vi "increment Modbus address.vi"(0 "available addresses":T1(array[cluster]), 1 "string length":i32, 5 "modbus type":T2, 7 "data type":T3) -> (4 "available addresses out":T1(array[cluster]), 6 "starting address":u16, 8 "subindex (bool)":i32)   [LabVIEW 2013, in "Modbus Module configuration.lvclass"]
uses:
  Modbus Module configuration.lvclass
  <vilib>/NI/Tag Bus/tag/Data Type.ctl
  module channel/data bank type.ctl
  <vilib>/NI/Tag Bus/tag/tag descriptor.lvclass
  module channel/Modbus Module Channel.lvclass
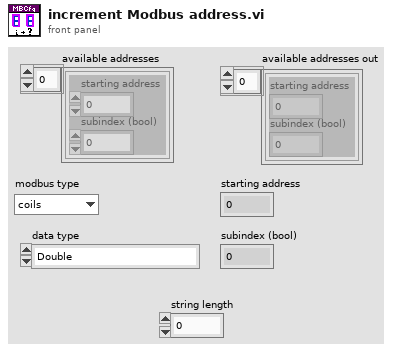
[diagram p1: front panel]
types:
  T1 = cluster{"starting address":u16, "subindex (bool)":i32}[]
  T2 = typedef "Modbus Module Channel.lvclass/data bank type.ctl" = enum16{"coils", "discrete inputs", "input registers", "holding registers"}
  T3 = typedef "tag bus.lvlib/tag descriptor.lvclass/Data Type.ctl" = enum16{"Double", "Single", "I64", "I32", "I16", "I8", "U64", "U32", "U16", "U8", "Boolean", "String", "Array of Double", "Array of Single", "Array of I64", "Array of I32", "Array of I16", "Array of I8", "Array of U64", "Array of U32", "Array of U16", "Array of U8", "Array of Boolean", "Array of String"}
  T4 = cluster{"starting address":u16, "subindex (bool)":i32}
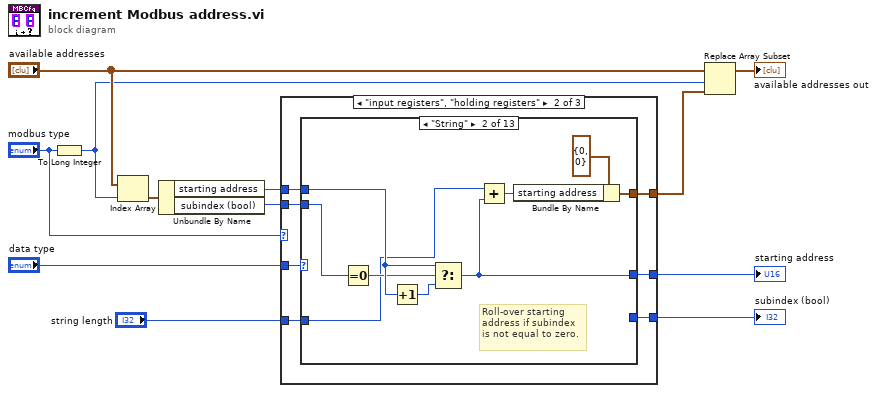
[diagram p0: block diagram]
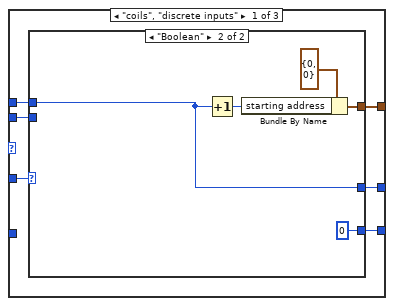
[diagram p2: hidden frame]
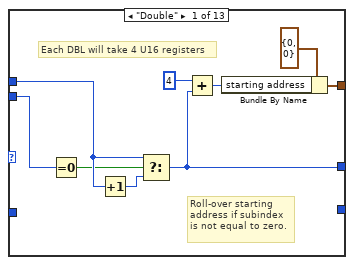
[diagram p4: hidden frame]
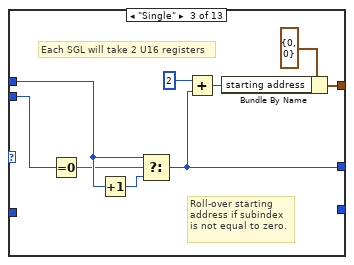
[diagram p5: hidden frame]
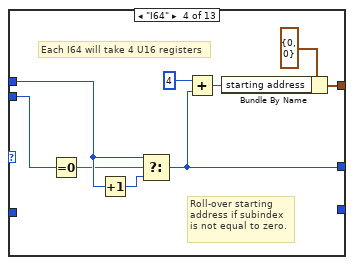
[diagram p6: hidden frame]
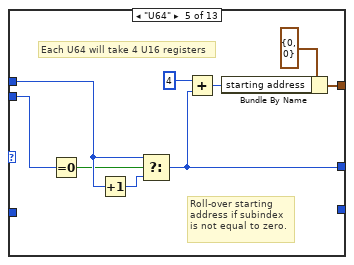
[diagram p7: hidden frame]
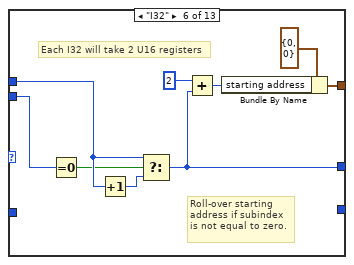
[diagram p8: hidden frame]
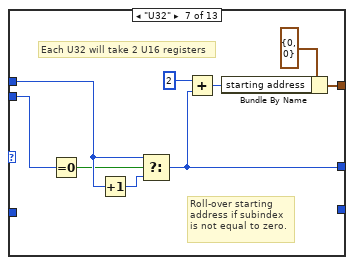
[diagram p9: hidden frame]
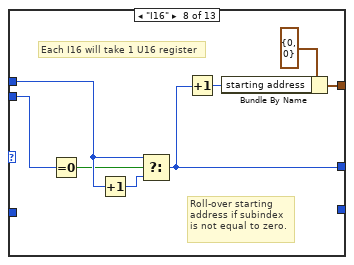
[diagram p10: hidden frame]
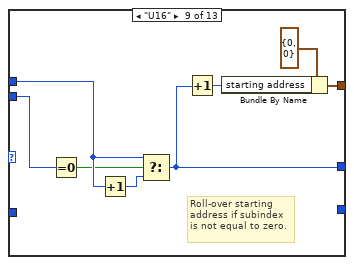
[diagram p11: hidden frame]
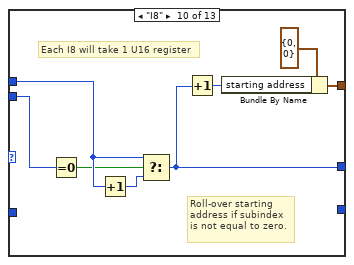
[diagram p12: hidden frame]
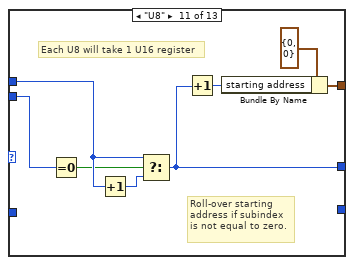
[diagram p13: hidden frame]
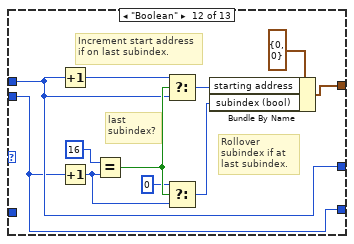
[diagram p14: hidden frame]
diagram:
  n1 = To Long Integer(number="modbus type") -> (32bit integer=w9:i32)
  n2 = Index Array(array="available addresses", index=w9) -> (element=w11:T4)
  n3 = Unbundle By Name(w11) -> ("starting address"=w5:u16, "subindex (bool)"=w8:i32)
  n4 = case shown="\"input registers\", \"holding registers\"" "modbus type" {
    tunnel: "data type" -> [w18 w30 _]
    tunnel: w8 -> [w17 w29 _]
    tunnel: [w16 w28 _] -> w6
    tunnel: w5 -> [w15 w27 _]
    tunnel: [w14 w26 _] -> w4
    tunnel: [w13 w25 _] -> w3
    tunnel: "string length" -> [_ w24 _]
    frame "coils", "discrete inputs" {
      n5 = case shown="\"Boolean\"" w18 {
        tunnel: w17 -> [_ _]
        tunnel: w15 -> [_ w19]
        tunnel: [_ w22] -> w16
        tunnel: [_ w19] -> w14
        tunnel: [_ 0 ("subindex (bool)")] -> w13
        frame Default {
        }
        frame "Boolean" {
          n6 = Increment(x=w19) -> (x+1=w21:u16)
          n7 = Bundle By Name(cluster=T4 {"starting address"=0, "subindex (bool)"=0} ("element"), "starting address"=w21) -> (w22:T4)
        }
      }
    }
    frame "input registers", "holding registers" {
      n8 = case shown="\"String\"" w30 {
        tunnel: w29 -> [w36 w46 w54 w63 w72 w81 w90 w99 w107 w115 w123 w126 _]
        tunnel: w27 -> [w35 w45 w53 w62 w71 w80 w89 w98 w106 w114 w122 w127 _]
        tunnel: [w38 w47 w56 w65 w74 w83 w92 w100 w108 w116 w124 w135 _] -> w28
        tunnel: [w32 w42 w50 w59 w68 w77 w86 w95 w103 w111 w119 w127 _] -> w26
        tunnel: [_ _ _ _ _ _ _ _ _ _ _ w126 _] -> w25
        tunnel: w24 -> [_ w40 _ _ _ _ _ _ _ _ _ _ _]
        frame "Double" {
          # "Each DBL will take 4 U16 registers"
          # "Roll-over starting\naddress if subindex\nis not equal to zero."
          n9 = Equal To 0?(x=w36) -> (x = 0?=w33:bool)
          n10 = Increment(x=w35) -> (x+1=w34:u16)
          n11 = Select(t=w35, s=w33, f=w34) -> (s? t:f=w32:u16)
          n12 = Add(x=u16 4, y=w32) -> (x+y=w31:u16)
          n13 = Bundle By Name(cluster=T4 {"starting address"=0, "subindex (bool)"=0} ("element"), "starting address"=w31) -> (w38:T4)
        }
        frame "String" {
          # "Roll-over starting\naddress if subindex\nis not equal to zero."
          n14 = Equal To 0?(x=w46) -> (x = 0?=w43:bool)
          n15 = Increment(x=w45) -> (x+1=w44:u16)
          n16 = Select(t=w45, s=w43, f=w44) -> (s? t:f=w42:u16)
          n17 = Add(x=w40, y=w42) -> (x+y=w41:i32)
          n18 = Bundle By Name(cluster=T4 {"starting address"=0, "subindex (bool)"=0} ("element"), "starting address"=w41) -> (w47:T4)
        }
        frame "Single" {
          # "Each SGL will take 2 U16 registers"
          # "Roll-over starting\naddress if subindex\nis not equal to zero."
          n19 = Equal To 0?(x=w54) -> (x = 0?=w51:bool)
          n20 = Increment(x=w53) -> (x+1=w52:u16)
          n21 = Select(t=w53, s=w51, f=w52) -> (s? t:f=w50:u16)
          n22 = Add(x=u16 2, y=w50) -> (x+y=w49:u16)
          n23 = Bundle By Name(cluster=T4 {"starting address"=0, "subindex (bool)"=0} ("element"), "starting address"=w49) -> (w56:T4)
        }
        frame "I64" {
          # "Each I64 will take 4 U16 registers"
          # "Roll-over starting\naddress if subindex\nis not equal to zero."
          n24 = Equal To 0?(x=w63) -> (x = 0?=w60:bool)
          n25 = Increment(x=w62) -> (x+1=w61:u16)
          n26 = Select(t=w62, s=w60, f=w61) -> (s? t:f=w59:u16)
          n27 = Add(x=u16 4, y=w59) -> (x+y=w58:u16)
          n28 = Bundle By Name(cluster=T4 {"starting address"=0, "subindex (bool)"=0} ("element"), "starting address"=w58) -> (w65:T4)
        }
        frame "U64" {
          # "Each U64 will take 4 U16 registers"
          # "Roll-over starting\naddress if subindex\nis not equal to zero."
          n29 = Equal To 0?(x=w72) -> (x = 0?=w69:bool)
          n30 = Increment(x=w71) -> (x+1=w70:u16)
          n31 = Select(t=w71, s=w69, f=w70) -> (s? t:f=w68:u16)
          n32 = Add(x=u16 4, y=w68) -> (x+y=w67:u16)
          n33 = Bundle By Name(cluster=T4 {"starting address"=0, "subindex (bool)"=0} ("element"), "starting address"=w67) -> (w74:T4)
        }
        frame "I32" {
          # "Each I32 will take 2 U16 registers"
          # "Roll-over starting\naddress if subindex\nis not equal to zero."
          n34 = Equal To 0?(x=w81) -> (x = 0?=w78:bool)
          n35 = Increment(x=w80) -> (x+1=w79:u16)
          n36 = Select(t=w80, s=w78, f=w79) -> (s? t:f=w77:u16)
          n37 = Add(x=u16 2, y=w77) -> (x+y=w76:u16)
          n38 = Bundle By Name(cluster=T4 {"starting address"=0, "subindex (bool)"=0} ("element"), "starting address"=w76) -> (w83:T4)
        }
        frame "U32" {
          # "Each U32 will take 2 U16 registers"
          # "Roll-over starting\naddress if subindex\nis not equal to zero."
          n39 = Equal To 0?(x=w90) -> (x = 0?=w87:bool)
          n40 = Increment(x=w89) -> (x+1=w88:u16)
          n41 = Select(t=w89, s=w87, f=w88) -> (s? t:f=w86:u16)
          n42 = Add(x=u16 2, y=w86) -> (x+y=w85:u16)
          n43 = Bundle By Name(cluster=T4 {"starting address"=0, "subindex (bool)"=0} ("element"), "starting address"=w85) -> (w92:T4)
        }
        frame "I16" {
          # "Each I16 will take 1 U16 register"
          # "Roll-over starting\naddress if subindex\nis not equal to zero."
          n44 = Equal To 0?(x=w99) -> (x = 0?=w96:bool)
          n45 = Increment(x=w98) -> (x+1=w97:u16)
          n46 = Select(t=w98, s=w96, f=w97) -> (s? t:f=w95:u16)
          n47 = Increment(x=w95) -> (x+1=w94:u16)
          n48 = Bundle By Name(cluster=T4 {"starting address"=0, "subindex (bool)"=0} ("element"), "starting address"=w94) -> (w100:T4)
        }
        frame "U16" {
          # "Roll-over starting\naddress if subindex\nis not equal to zero."
          n49 = Equal To 0?(x=w107) -> (x = 0?=w104:bool)
          n50 = Increment(x=w106) -> (x+1=w105:u16)
          n51 = Select(t=w106, s=w104, f=w105) -> (s? t:f=w103:u16)
          n52 = Increment(x=w103) -> (x+1=w102:u16)
          n53 = Bundle By Name(cluster=T4 {"starting address"=0, "subindex (bool)"=0} ("element"), "starting address"=w102) -> (w108:T4)
        }
        frame "I8" {
          # "Each I8 will take 1 U16 register"
          # "Roll-over starting\naddress if subindex\nis not equal to zero."
          n54 = Equal To 0?(x=w115) -> (x = 0?=w112:bool)
          n55 = Increment(x=w114) -> (x+1=w113:u16)
          n56 = Select(t=w114, s=w112, f=w113) -> (s? t:f=w111:u16)
          n57 = Increment(x=w111) -> (x+1=w110:u16)
          n58 = Bundle By Name(cluster=T4 {"starting address"=0, "subindex (bool)"=0} ("element"), "starting address"=w110) -> (w116:T4)
        }
        frame "U8" {
          # "Each U8 will take 1 U16 register"
          # "Roll-over starting\naddress if subindex\nis not equal to zero."
          n59 = Equal To 0?(x=w123) -> (x = 0?=w120:bool)
          n60 = Increment(x=w122) -> (x+1=w121:u16)
          n61 = Select(t=w122, s=w120, f=w121) -> (s? t:f=w119:u16)
          n62 = Increment(x=w119) -> (x+1=w118:u16)
          n63 = Bundle By Name(cluster=T4 {"starting address"=0, "subindex (bool)"=0} ("element"), "starting address"=w118) -> (w124:T4)
        }
        frame "Boolean" {
          # "Increment start address\nif on last subindex."
          # "Rollover subindex if at last subindex."
          # "last\nsubindex?"
          n64 = Increment(x=w127) -> (x+1=w129:u16)
          n65 = Increment(x=w126) -> (x+1=w128:i32)
          n66 = Equal?(x=16, y=w128) -> (x = y?=w133:bool)
          n67 = Select(t=w129, s=w133, f=w127) -> (s? t:f=w131:u16)
          n68 = Select(t=0, s=w133, f=w128) -> (s? t:f=w130:i32)
          n69 = Bundle By Name(cluster=T4 {"starting address"=0, "subindex (bool)"=0} ("element"), "starting address"=w131, "subindex (bool)"=w130) -> (w135:T4)
        }
        frame Default {
        }
      }
    }
    frame Default {
    }
  }
  "subindex (bool)" <- w3
  "starting address" <- w4
  n70 = Replace Array Subset(array="available addresses", new element=w6, index=w9) -> (→"available addresses out":T1)
